vi "STS_Get_Calibrated_IL.vi"(8 "错误输入（无错误）":errorcluster, 11 ".NET引用句柄输入":refnum<k24>) -> (0 "error out":errorcluster, 1 "calibratedIL":sgl[][](array[numeric]), 3 "引用输出":refnum<k24>)   [LabVIEW 2017]
doc: "Process ranges merge"
uses:
  D:/test/PDLSTS/LV_PDL_Sample/DLL/STSProcess.dll
  DLL/STSProcess.dll
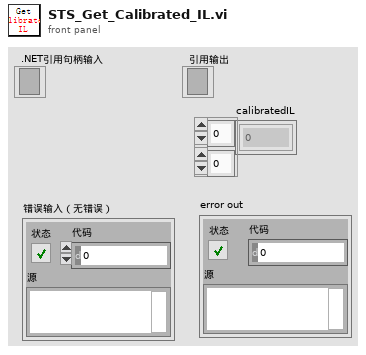
[diagram p1: front panel]
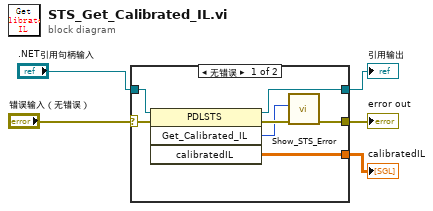
[diagram p0: block diagram]
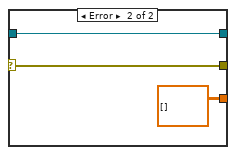
[diagram p2: hidden frame]
diagram:
  n1 = case shown="无错误" "错误输入（无错误）" {
    selector: "错误输入（无错误）" -> [w11 w15]
    tunnel: ".NET引用句柄输入" -> [w12 w14]
    tunnel: [w8 w15] -> w3
    tunnel: [w7 w14] -> w2
    tunnel: [w6 sgl[][] [] ("calibratedIL")] -> w1
    frame No Error {
      n2 = invoke class="PDLSTS" method="Get_Calibrated_IL"(reference=w12, error in=w11) -> (reference out=w7:refnum<k24>, error out=w10:errorcluster, "Get_Calibrated_IL"=w9:i32, "calibratedIL"=w6:sgl[][])  [unwired: 2 in]
      n3 = call "Show_STS_Error.vi"("error in (no error)"=w10, "Error"=w9) -> ("error out"=w8:errorcluster)  [unwired: 9 in]
    }
    frame Error {
    }
  }
  "error out" <- w3
  "引用输出" <- w2
  "calibratedIL" <- w1
